vi "visible-frame-case-sequence.vi"   [LabVIEW 2025]
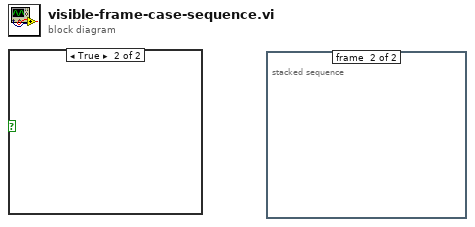
[diagram p0: block diagram]
diagram:
  n1 = case shown="True" {
    selector: _ -> [_ _]
    frame False {
    }
    frame True {
    }
  }
  n2 = stacked-sequence {
    frame #0 {
    }
    frame #1 {
    }
  }
